vi "createElements.vi"(8 "error in (no error)":errorcluster, 11 "Topic in":refnum<class "Topic.lvclass">) -> (0 "error out":errorcluster, 3 "Topic out":refnum<class "Topic.lvclass">)   [LabVIEW 2012, in "Topic.lvclass"]
uses:
  Topic.lvclass
  Topic.lvclass/Topic.ctl
  Element/Element.lvclass
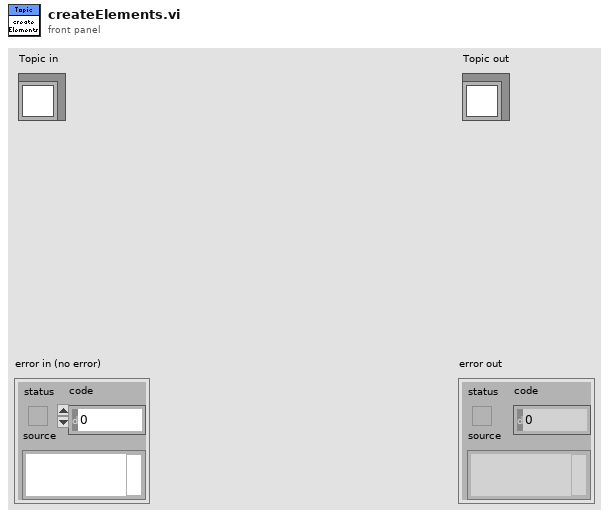
[diagram p1: front panel]
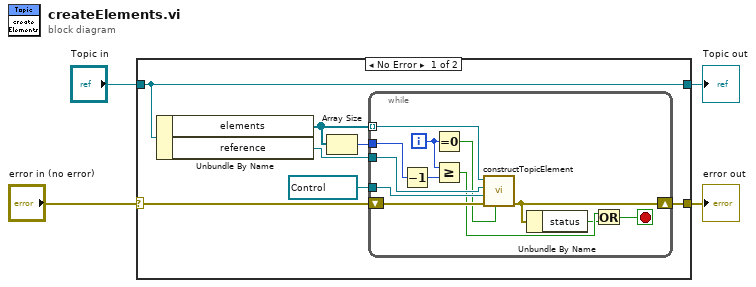
[diagram p0: block diagram]
diagram:
  n1 = case shown="No Error" "error in (no error)" {
    selector: "error in (no error)" -> [w9 w25]
    tunnel: [w8 w25] -> w3
    tunnel: [w11 w24] -> w1
    tunnel: "Topic in" -> [w11 w24]
    frame No Error {
      n2 = Unbundle By Name(w11) -> ("elements"=w6:refnum<class "Element.lvclass">[], "reference"=w10:refnum<vi>)
      n3 = Array Size(array=w6) -> (size(s)=w5:i32)
      n4 = while {
        tunnel: w6 -> [w23] mode=indexing
        tunnel: w10 -> [w22]
        shift-right: [w14] -> w8
        shift-left: w9 -> [w21]
        tunnel: refnum<vi> refnum ("prevObjRef") -> [w20]
        tunnel: w5 -> [w16]
        i -> [w17]
        stop <- w12 stop-if-true
        n5 = Decrement(x=w16) -> (x-1=w18:i32)
        n6 = Equal To 0?(x=w17) -> (x = 0?=w19:bool)
        n7 = Greater Or Equal?(x=w17, y=w18) -> (x >= y?=w15:bool)
        n8 = call "constructTopicElement.vi"("firstItem? (F)"=w19, "error in (no error)"=w21, "prevObjRef"=w20, "clusterInfo.reference"=w22, "Element in"=w23) -> ("error out"=w14:errorcluster)  [unwired: 5 in, 1 out]
        n9 = Unbundle By Name(w14) -> ("status"=w13:bool)
        n10 = Or(x=w15, y=w13) -> (x .or. y?=w12:bool)
      }
    }
    frame Error {
    }
  }
  "error out" <- w3
  "Topic out" <- w1
